vi "closeCOMport.vi"(0 "COM port":refnum<visa-resource-name>) -> ()   [LabVIEW 2015]
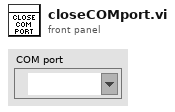
[diagram p1: front panel]
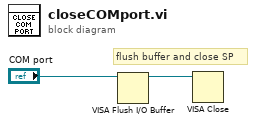
[diagram p0: block diagram]
diagram:
  # "flush buffer and close SP"
  n1 = VISA Flush I/O Buffer(VISA resource name="COM port") -> (VISA resource name out=w2:refnum<visa-resource-name>)  [unwired: 2 in, 1 out]
  n2 = VISA Close(VISA resource name=w2) -> ()  [unwired: 1 in, 1 out]
